vi "set_refnum.vi"(8 "error in (no error)":errorcluster, 10 "ref":u64, 11 "Headers in":refnum<class "Headers.lvclass">) -> (0 "error out":errorcluster, 3 "Headers out":refnum<class "Headers.lvclass">)   [LabVIEW 2020, in "reqwest.lvlib" / "Headers.lvclass"]
uses:
  Headers.lvclass
  Headers.lvclass/Headers.ctl
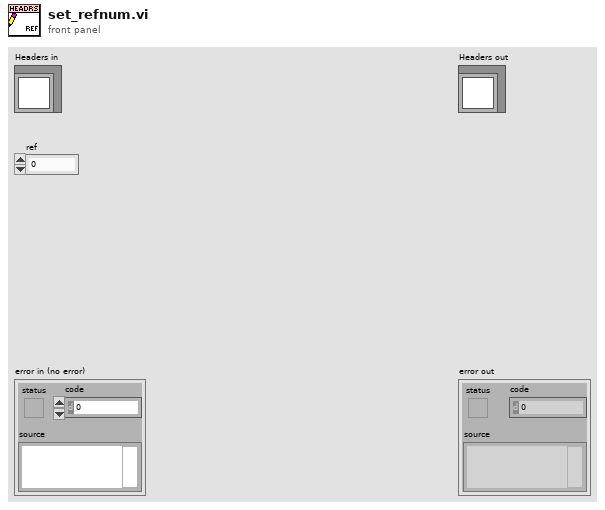
[diagram p1: front panel]
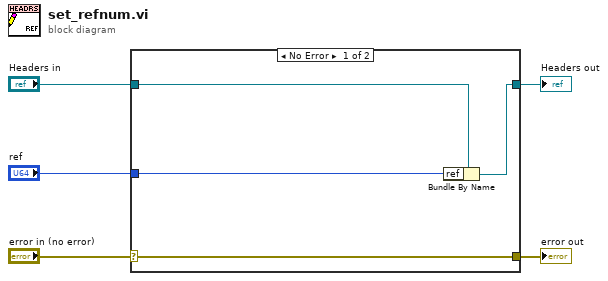
[diagram p0: block diagram]
diagram:
  n1 = case shown="No Error" "error in (no error)" {
    selector: "error in (no error)" -> [w9 w10]
    tunnel: [w9 w10] -> w4
    tunnel: [w7 w11] -> w2
    tunnel: "Headers in" -> [w8 w11]
    tunnel: "ref" -> [w6 _]
    frame No Error {
      n2 = Bundle By Name(cluster=w8, "ref"=w6) -> (w7:refnum<class "Headers.lvclass">)
    }
    frame Error {
    }
  }
  "error out" <- w4
  "Headers out" <- w2
